vi "Create Database.vi"() -> ()   [LabVIEW 2014]
doc: "<B>Copyright</B>: (c) 2015 MHWirth. All rights reserved.\n\nCreates a database for the variables on one deployed process. \n\n<B>need to extend</B>"
uses:
  <vilib>/Utility/file.llb/Write To Spreadsheet File (string).vi
panel:
  in  "file path (dialog if empty)":path=path "C:/Ehsan Temp Folder/TFS/LV/Topside Manager/support/support/SVname.txt"
  out "Number of Variables":i32
  in  "container refnum in":refnum<k21>="ni.var.psp://localhost"
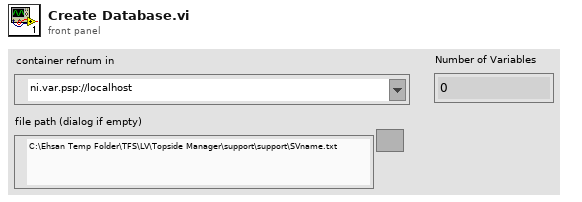
[diagram p1: front panel]
types:
  T1 = cluster{"Number of Variables":i32, "Variable/Parent Name array":string[][], "URL array":string[], "Type array":string[]}
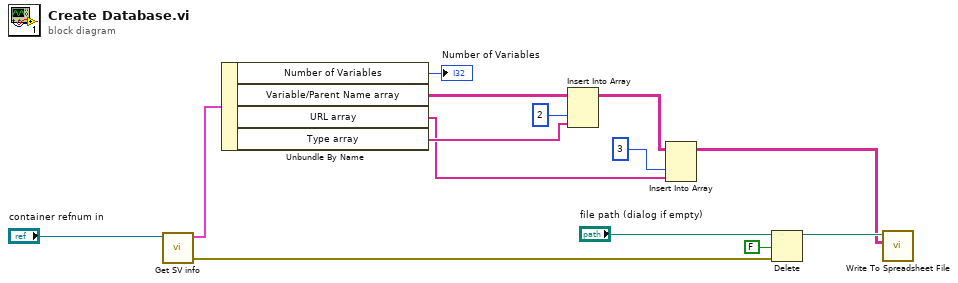
[diagram p0: block diagram]
diagram:
  n1 = call "Get SV info.vi"("container refnum in"="container refnum in") -> ("Error Out"=w10:errorcluster, "Deployed Shared Variable Information"=w1:T1)  [unwired: 8 in, 1 out]
  n2 = Unbundle By Name(w1) -> ("Number of Variables"=→"Number of Variables":i32, "Variable/Parent Name array"=w4:string[][], "URL array"=w2:string[], "Type array"=w7:string[])
  n3 = Insert Into Array(array=w4, index (col)=2 ("disabled index (col)"), new element=w7) -> (w3:string[][])  [unwired: 1 in]
  n4 = Insert Into Array(array=w3, index (col)=3 ("disabled index (col)"), new element=w2) -> (w5:string[][])  [unwired: 1 in]
  n5 = Delete(path (use dialog)="file path (dialog if empty)", confirm (F)=FALSE, error in=w10) -> (deleted path=w12:path)  [unwired: 2 in, 2 out]
  n6 = call-poly <vilib>:"Write To Spreadsheet File.vi"("2D data"=w5, "file path (dialog if empty)"=w12) -> ()  [unwired: 6 in, 1 out]
